vi "zmq curve public.vi"(8 "error in (no error)":errorcluster, 10 "z85_secret_key_":string, 11 "z85_public_key_":string) -> (0 "error out":errorcluster, 2 "function return":i32, 3 "z85_public_key_ out":string)   [LabVIEW 2025, in "libzmq-v143-mt-4_3_6.lvlib"]
doc: "ZMQ_EXPORT int zmq_curve_public (char *z85_public_key_,\n const char *z85_secret_key_);"
uses:
  libzmq-v143-mt-4_3_6.lvlib
  LV/LibZMQ/libzmq/lv_x86/bin/Release/libzmq-v143-mt-4_3_6.dll
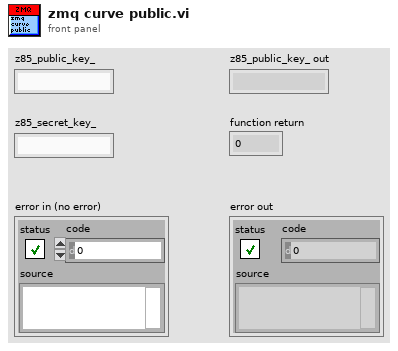
[diagram p1: front panel]
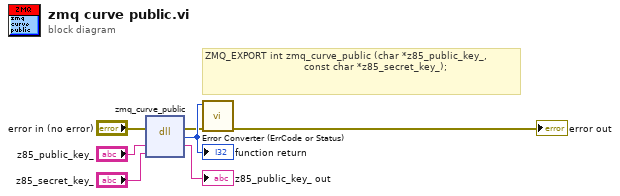
[diagram p0: block diagram]
diagram:
  # "ZMQ_EXPORT int zmq_curve_public (char *z85_public_key_,\n                                 const char *z85_secret_key_);"
  n1 = dll-call lib="C:/LV/LibZMQ/libzmq/lv_x86/bin/Release/libzmq-v143-mt-4_3_6.*" fn="zmq_curve_public"(error in="error in (no error)", "z85_public_key_"="z85_public_key_", "z85_secret_key_"="z85_secret_key_") -> (error out=w2:errorcluster, w7:i32, "z85_public_key_"=→"z85_public_key_ out":string)  [unwired: 3 in, 1 out]
  "function return" <- w7
  n2 = call "Error Converter (ErrCode or Status).vi"("error in (no error)"=w2, "error code"=w7) -> ("error out"=→"error out":errorcluster)  [unwired: 9 in]
